vi "run.vi"(7 "execution system":T1=enum."standard", 8 "error in":errorcluster, 9 "results reporter":refnum<class "results reporter.lvclass">, 10 "task":refnum<class "task.lvclass">, 11 "thread pool in":refnum<class "thread pool.lvclass">) -> (0 "error out":errorcluster, 3 "thread pool out":refnum<class "thread pool.lvclass">)   [LabVIEW 2015, in "thread pool.lvclass"]
uses:
  thread pool.lvclass
  task/task.lvclass
  execution system.ctl
  results reporter/results reporter.lvclass
  task/strict executor reference.ctl
  thread pool.lvclass/thread pool.ctl
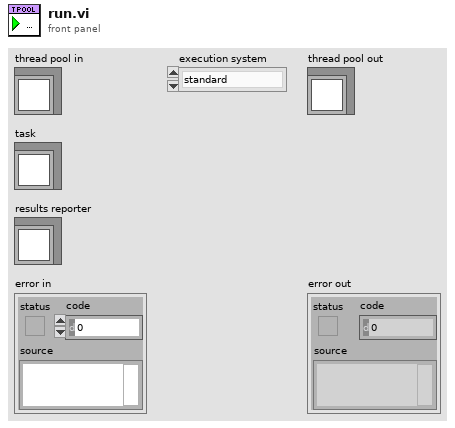
[diagram p1: front panel]
types:
  T1 = typedef "thread pool.lvclass/execution system.ctl" = enum32{"user interface", "standard", "instrument i/o", "data acquisition", "other 1", "other 2"}
  T2 = typedef "thread pool.lvclass/strict executor reference.ctl" = refnum<vi>
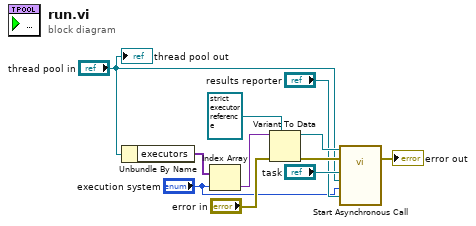
[diagram p0: block diagram]
diagram:
  n1 = Unbundle By Name("thread pool in") -> ("executors"=w8:variant[])
  n2 = Index Array(array=w8, index="execution system") -> (element=w6:variant)
  n3 = Variant To Data(error in="error in", type=T2 refnum ("executor reference"), Variant=w6) -> (data=w4:T2, error out=w7:errorcluster)
  n4 = call-by-ref "Start Asynchronous Call"(reference=w4, error in=w7, "results reporter"="results reporter", "execution system"="execution system", "thread pool"="thread pool in", "task"="task") -> (error out=→"error out":errorcluster)  [unwired: 8 in, 1 out]
  "thread pool out" <- "thread pool in"
